vi "index_array_many.vi"(1 "Lines of Array to grab":i16[](array[numeric]), 2 "String Array Input":string[](array[string])) -> (0 "Output array":string[](array[string]))   [LabVIEW 2014]
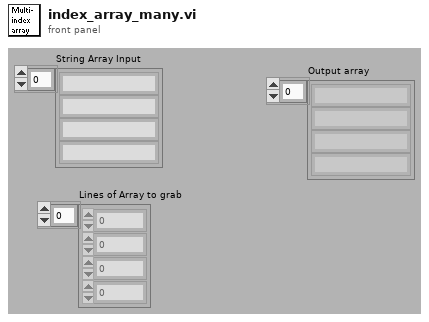
[diagram p1: front panel]
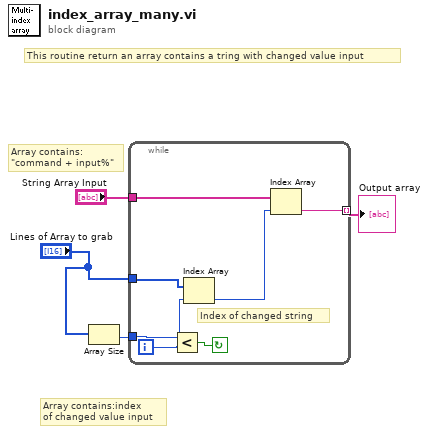
[diagram p0: block diagram]
diagram:
  # "This routine return an array contains a tring with changed value input"
  # "Array contains:index\nof changed value input"
  # "Array contains:\n\"command + input%\""
  n1 = Array Size(array="Lines of Array to grab") -> (size(s)=w4:i32)
  n2 = while {
    tunnel: w4 -> [w11]
    tunnel: "Lines of Array to grab" -> [w9]
    tunnel: "String Array Input" -> [w6]
    tunnel: [w5] -> w1 mode=indexing
    i -> [w8]
    stop <- w10 continue-if-true
    # "Index of changed string"
    n3 = Less?(x=w11, y=w8) -> (x < y?=w10:bool)
    n4 = Index Array(array=w9, index=w8) -> (element=w7:i16)
    n5 = Index Array(array=w6, index=w7) -> (element=w5:string)
  }
  "Output array" <- w1
